vi "EOL Oscope AI Hall Buffer.vi"(8 "Data Write(Single)":dbl[](array[numeric]), 9 "Buffer Size (seconds/2500)":i32=5000, 11 "Mode":enum16{"Initialize", "Read", "Write"}(ring)=enum."Read") -> (2 "Data Read (Single)":sgl[](array[numeric]) format="%.2f")   [LabVIEW 2018]
doc: "This VI is used in many locations throughout the program as a data buffer. It serves mainly two purposes. In alarms and logging, the DAQ data, whether scaled or voltage, is entered into the buffer. In other parts of the program, data is read from the buffer. Its length is based on the # of samples it was initialized to.\n\nA read will always return the latest data of the size requested."
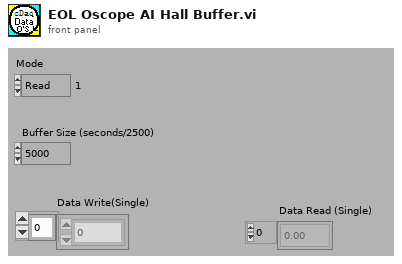
[diagram p1: front panel]
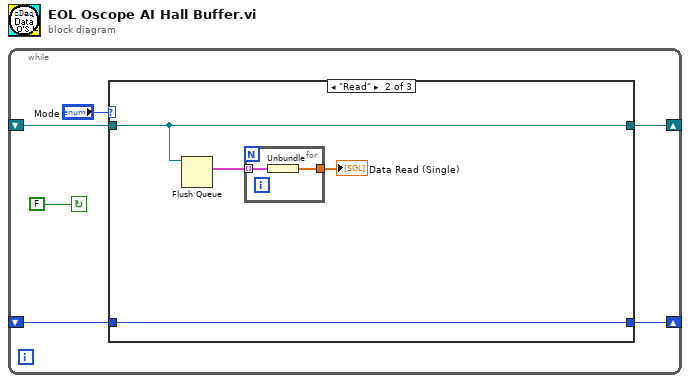
[diagram p0: block diagram]
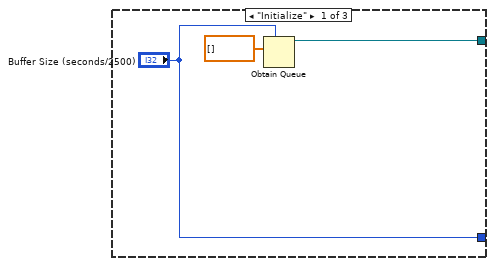
[diagram p2: hidden frame]
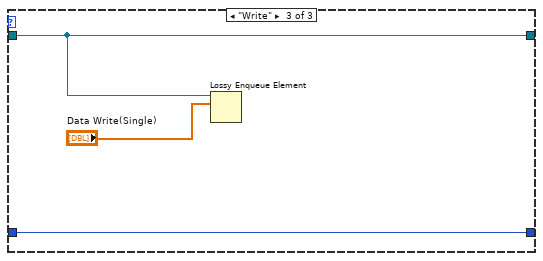
[diagram p3: hidden frame]
diagram:
  n1 = while {
    shift-left: _ -> [w5]
    shift-right: [w4] -> _
    shift-right: [w2] -> _
    shift-left: _ -> [w1]
    stop <- FALSE continue-if-true
    n2 = case shown="\"Read\"" "Mode" {
      tunnel: ["Buffer Size (seconds/2500)" w13 w18] -> w4
      tunnel: w5 -> [_ w13 w18]
      tunnel: [w8 w12 w17] -> w2
      tunnel: w1 -> [_ w12 w17]
      frame "Initialize" {
        n3 = Obtain Queue(max queue size (-1, unlimited)="Buffer Size (seconds/2500)", element data type=sgl[] []) -> (queue out=w8:refnum<queue>)  [unwired: 3 in, 2 out]
      }
      frame "Read" {
        n4 = Flush Queue(queue=w12) -> (remaining elements=w11:cluster{sgl[]}[])  [unwired: 1 in, 2 out]
        n5 = for {
          tunnel: w11 -> [w15] mode=indexing
          tunnel: [w14] -> w10
          n6 = Unbundle(w15) -> (w14:sgl[])
        }
        "Data Read (Single)" <- w10
      }
      frame "Write" {
        n7 = Lossy Enqueue Element(queue=w17, element="Data Write(Single)") -> ()  [unwired: 1 in, 4 out]
      }
    }
  }
